vi "Music Visualizer Template LV2014.vi"() -> ()   [LabVIEW 2015]
uses:
  <vilib>/Analysis/3filter.llb/Filter Passband Type.ctl
  <vilib>/sound2/lvsound2.llb/Sampling Mode.ctl
  <vilib>/sound2/lvsound2.llb/Sound Output Write (DBL).vi
  <vilib>/Analysis/3filter.llb/Butterworth Filter (DBL).vi
  <vilib>/sound2/lvsound2.llb/Sound File Read (DBL).vi
  <vilib>/sound2/lvsound2.llb/Sound File Read Open.vi
  <vilib>/sound2/lvsound2.llb/Sound File Info (path).vi
  <vilib>/measure/maspectr.llb/FFT Power Spectrum and PSD for 1 Chan.vi
  <vilib>/measure/NI_MAPro.lvlib
  <vilib>/Analysis/NI_AALBase.lvlib
panel:
  out "Low Cutoff Freq, Hz":u32
  out "High Cutoff Freq, Hz":u32
  out "Filter Error!":bool
  in  "Filter Bands ,Hz":cluster{dbl, dbl}(slide)={22000.0, 10.0} scale=10.0..22000.0
  in  "Filter Type":T1=enum."Bandpass"
  out "Power Spectrum":waveform(dbl)(graph)
  out "digital spectrum":dbl[](array[slide]) scale=-42.0..6.0
  out "VU":dbl(knob) scale=-42.0..6.0
  out "Waveform":waveform(dbl)[](graph)
  in  "Stop":bool
  in  "Buffer Size (samples)":i32=2048
  in  "Music File":path=path "C:/Users/londov/Documents/code/labview/audio visualizer/audio/dupstep.wav"
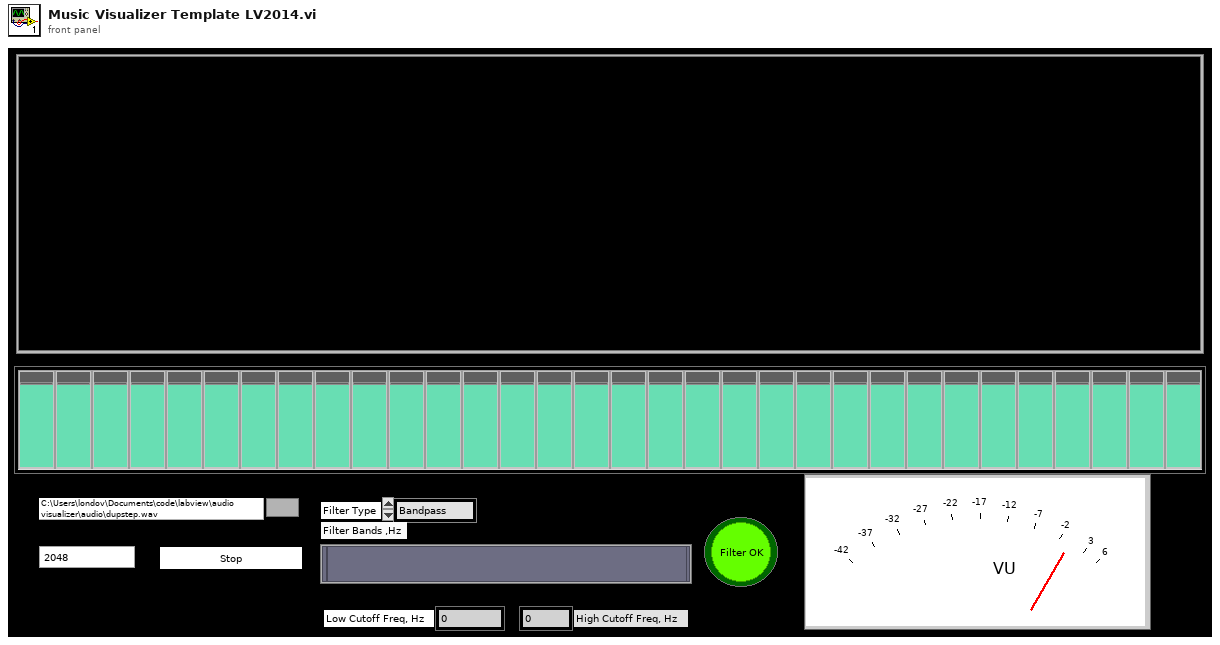
[diagram p1: front panel]
types:
  T1 = typedef "NI_AALBase.lvlib/Filter Passband Type.ctl" = enum32{"Lowpass", "Highpass", "Bandpass", "Bandstop"}
  T2 = typedef "Sampling Mode.ctl" = i32
  T3 = typedef "Sound Data Format.ctl" = cluster{"sample rate (S/s)":dbl, "number of channels":i32, "bits per sample":i32}
  T4 = typedef "Sound Output Task ID.ctl" = u32
  T5 = typedef "Sound File Refnum.ctl" = refnum<file>
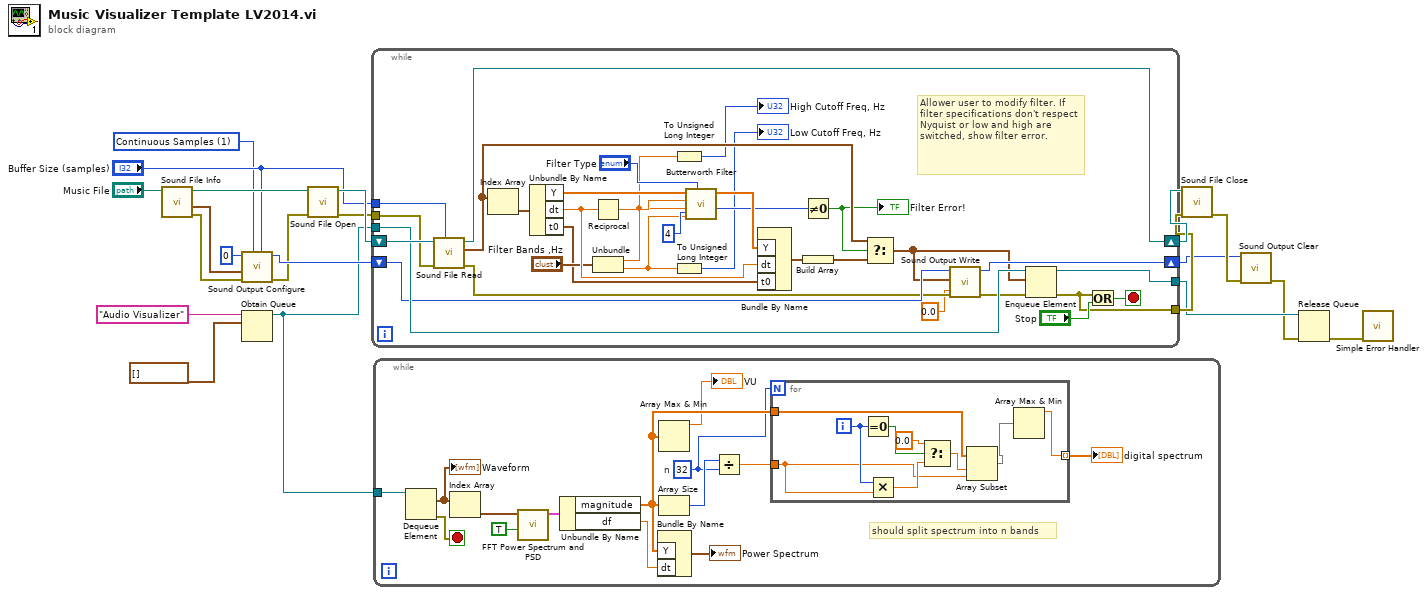
[diagram p0: block diagram]
diagram:
  w1 = T2 1 items=["Finite Samples", "Continuous Samples"] ("sample mode")
  n1 = call-poly <vilib>:"Sound File Info.vi"("path"="Music File") -> ("error out"=w4:errorcluster, "sound format"=w11:T3, "path out"=w14:path)  [unwired: 7 in, 1 out]
  n2 = call <vilib>:"Sound Output Configure.vi"("number of samples/ch"="Buffer Size (samples)", "sample mode"=w1, "error in (no error)"=w4, "sound format"=w11, "device ID"=u32 0) -> ("error out"=w3:errorcluster, "task ID"=w9:T4)  [unwired: 5 in]
  n3 = Obtain Queue(name (unnamed)="Audio Visualizer", element data type=waveform(dbl)[] [] ("data")) -> (queue out=w8:refnum<queue>)  [unwired: 3 in, 2 out]
  n4 = call-poly <vilib>:"Sound File Open.vi"("error in (no error)"=w3, "path"=w14) -> ("error out"=w19:errorcluster, "sound file refnum"=w21:T5)  [unwired: 8 in]
  n5 = while {
    tunnel: "Buffer Size (samples)" -> [w53]
    shift-right: [w52] -> w20
    shift-left: w21 -> [w54]
    tunnel: w19 -> [w51]
    tunnel: [w47] -> w18
    tunnel: w8 -> [w48]
    tunnel: [w46] -> w17
    shift-right: [w42] -> w5
    shift-left: w9 -> [w45]
    stop <- w50 stop-if-true
    # "Allower user to modify filter. If filter specifications don't respect Nyquist or low and high are switched, show filter error."
    n6 = call-poly <vilib>:"Sound File Read.vi"("number of samples/ch (-1: all)"=w53, "error in (no error)"=w51, "sound file refnum"=w54) -> ("error out"=w44:errorcluster, "data"=w30:waveform(dbl)[], "sound file refnum out"=w52:T5)  [unwired: 4 in, 2 out]
    n7 = Index Array(array=w30) -> (element=w37:waveform(dbl))  [unwired: 1 in]
    n8 = Unbundle By Name(w37) -> ("Y"=w38:dbl[], "dt"=w34:dbl, "t0"=w27:timestamp)
    n9 = Reciprocal(x=w34) -> (1/x=w32:dbl)
    n10 = Unbundle("Filter Bands ,Hz") -> (w25:dbl, w24:dbl)
    n11 = To Unsigned Long Integer(number=w25) -> (unsigned 32bit integer=→"High Cutoff Freq, Hz":u32)
    n12 = To Unsigned Long Integer(number=w24) -> (unsigned 32bit integer=→"Low Cutoff Freq, Hz":u32)
    n13 = call-poly <vilib>:"Butterworth Filter.vi"("order"=4, "filter type"="Filter Type", "low cutoff freq: fl"=w24, "high cutoff freq: fh"=w25, "sampling freq: fs"=w32, "X"=w38) -> ("error"=w31:i32, "Filtered X"=w36:dbl[])  [unwired: 2 in]
    n14 = Bundle By Name("Y"=w36, "dt"=w34, "t0"=w27) -> (w35:waveform(dbl))  [unwired: 1 in]
    n15 = Not Equal To 0?(x=w31) -> (x != 0?=w26:bool)
    "Filter Error!" <- w26
    n16 = Build Array(w35) -> (w29:waveform(dbl)[])
    n17 = Select(t=w30, s=w26, f=w29) -> (s? t:f=w28:waveform(dbl)[])
    n18 = call-poly <vilib>:"Sound Output Write.vi"("timeout (sec)"=0.0, "error in (no error)"=w44, "data"=w28, "task ID"=w45) -> ("error out"=w43:errorcluster, "task ID out"=w42:T4)  [unwired: 6 in]
    n19 = Enqueue Element(queue=w48, element=w28, error in (no error)=w43) -> (queue out=w46:refnum<queue>, error out=w47:errorcluster)  [unwired: 1 in, 1 out]
    n20 = Or(x=w47, y="Stop") -> (x .or. y?=w50:bool)
  }
  n21 = while {
    tunnel: w8 -> [w68]
    stop <- w67 stop-if-true
    w57 = 32  # n
    # "should split spectrum into n bands"
    n22 = Dequeue Element(queue=w68) -> (element=w66:waveform(dbl)[], error out=w67:errorcluster)  [unwired: 2 in, 2 out]
    "Waveform" <- w66
    n23 = Index Array(array=w66) -> (element=w65:waveform(dbl))  [unwired: 1 in]
    n24 = call-poly <vilib>:"FFT Power Spectrum and PSD.vi"("dB On (F)"=TRUE, "time signal"=w65) -> ("Power Spectrum / PSD"=w63:cluster{"f0":dbl, "df":dbl, "magnitude":dbl[]})  [unwired: 6 in, 3 out]
    n25 = Unbundle By Name(w63) -> ("magnitude"=w58:dbl[], "df"=w62:dbl)
    n26 = Bundle By Name("Y"=w58, "dt"=w62) -> (→"Power Spectrum":waveform(dbl))  [unwired: 1 in]
    n27 = Array Max & Min(array=w58) -> (max value=→"VU":dbl)  [unwired: 3 out]
    n28 = Array Size(array=w58) -> (size(s)=w60:i32)
    n29 = Divide(x=w60, y=w57) -> (x/y=w59:dbl)
    n30 = for {
      N: w57 -> [_]
      tunnel: w59 -> [w71]
      tunnel: w58 -> [w77]
      tunnel: [w69] -> w55 mode=indexing
      i -> [w74]
      n31 = Equal To 0?(x=w74) -> (x = 0?=w76:bool)
      n32 = Multiply(x=w74, y=w71) -> (x*y=w73:dbl)
      n33 = Select(t=0.0, s=w76, f=w73) -> (s? t:f=w72:dbl)
      n34 = Array Subset(array=w77, index=w72, length=w71) -> (w70:dbl[])
      n35 = Array Max & Min(array=w70) -> (max value=w69:dbl)  [unwired: 3 out]
    }
    "digital spectrum" <- w55
  }
  n36 = call <vilib>:"Sound File Close.vi"("error in (no error)"=w18, "sound file refnum"=w20) -> ("error out"=w7:errorcluster)  [unwired: 9 in]
  n37 = call <vilib>:"Sound Output Clear.vi"("error in (no error)"=w7, "task ID"=w5) -> ("error out"=w6:errorcluster)  [unwired: 9 in]
  n38 = Release Queue(queue=w17, error in (no error)=w6) -> (error out=w16:errorcluster)  [unwired: 1 in, 2 out]
  n39 = call <vilib>:"Simple Error Handler.vi"("error in (no error)"=w16) -> ()  [unwired: 4 in, 5 out]
